vi "FTW-CodeGen-SetConstantValue.vi"(0 "GObject to Traverse":refnum<vi>, 5 "Constant Label":string="@FTW-CodeGen", 7 "Value":variant, 11 "error in":errorcluster) -> (15 "error out":errorcluster)   [LabVIEW 2014]
panel:
  # "Inputs"
  # "Outputs"
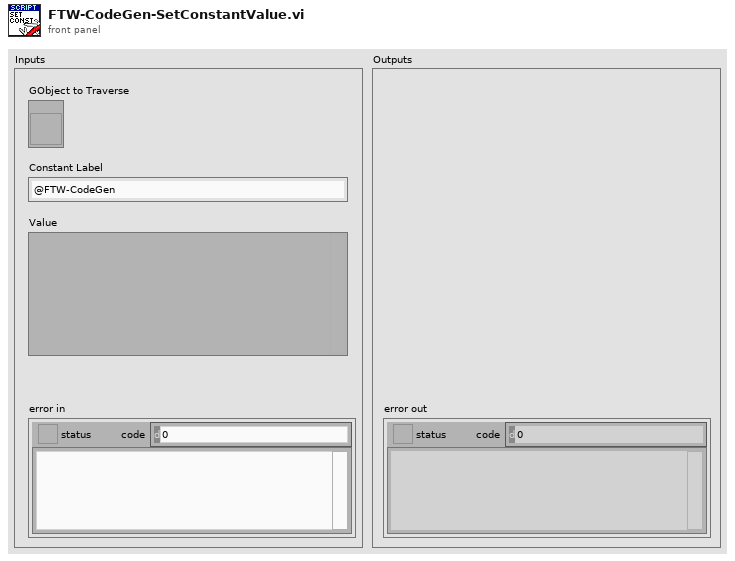
[diagram p1: front panel]
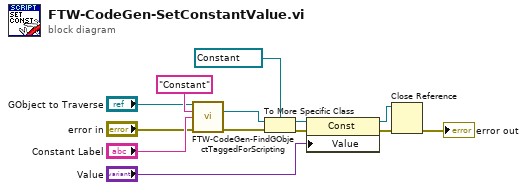
[diagram p0: block diagram]
diagram:
  n1 = call "FTW-CodeGen-FindGObjectTaggedForScripting.vi"("GObject to Traverse"="GObject to Traverse", "Class Name"="Constant", "Label Prefix to uniquely identify node"="Constant Label", "error in"="error in") -> ("GObject"=w12:refnum<vi>, "error out"=w11:errorcluster)  [unwired: 10 in]
  n2 = To More Specific Class(target class=refnum<vi> refnum ("Object"), reference=w12, error in=w11) -> (specific class reference=w10:refnum<vi>, error out=w9:errorcluster)
  n3 = property class="Const"(reference=w10, error in=w9, "Value"="Value") -> (reference out=w7:refnum<vi>, error out=w6:errorcluster)
  n4 = Close Reference(reference=w7, error in (no error)=w6) -> (error out=→"error out":errorcluster)
